vi "LoadDefaults.vi"(8 "Error In":errorcluster, 11 "Thorlabs In":refnum<class "Thorlabs.lvclass">) -> (0 "Error Out":errorcluster, 3 "Thorlabs Out":refnum<class "Thorlabs.lvclass">)   [LabVIEW 2018, in "Thorlabs.lvlib" / "Thorlabs.lvclass"]
doc: "This VI resets the Device to its defaults.\n\nCreator: Slade Jeppesen\nCreated Date: 09/29/20"
uses:
  Thorlabs.lvclass
  Thorlabs.lvclass/Thorlabs.ctl
  C:/AME Test Engineering/LabVIEW/PPLs/Axis/DLLs/ThorLabs.MotionControl.KCube.DCServoCLI.dll
  PPLs/Axis/DLLs/ThorLabs.MotionControl.KCube.DCServoCLI.dll
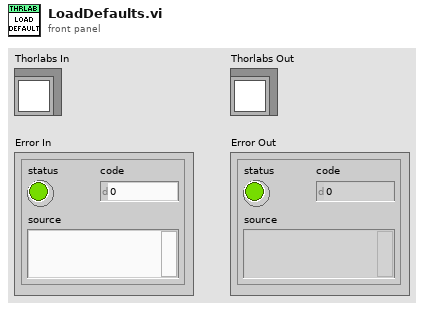
[diagram p1: front panel]
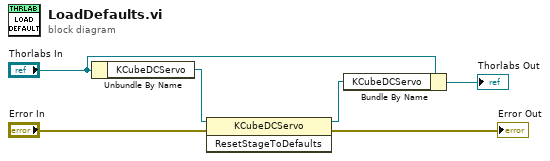
[diagram p0: block diagram]
diagram:
  n1 = Unbundle By Name("Thorlabs In") -> ("KCubeDCServo"=w6:refnum<k24>)
  n2 = invoke class="KCubeDCServo" method="ResetStageToDefaults"(reference=w6, error in="Error In") -> (reference out=w3:refnum<k24>, error out=→"Error Out":errorcluster)  [unwired: 1 in, 1 out]
  n3 = Bundle By Name(cluster="Thorlabs In", "KCubeDCServo"=w3) -> (→"Thorlabs Out":refnum<class "Thorlabs.lvclass">)
